vi "Global Stop Program.vi"() -> ()   [LabVIEW 2014]
panel:
  out "Global Stop Program":bool
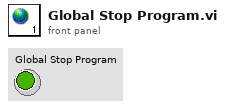
[diagram p1: front panel]
diagram:
